vi "uploadSaved.vi"(8 "error in":errorcluster, 11 "Path":path) -> (0 "error out":errorcluster)   [LabVIEW 2024]
uses:
  session.vi
  <vilib>/httpClient/POSTFile.vi
  <vilib>/httpClient/LabVIEWHTTPClient.lvlib
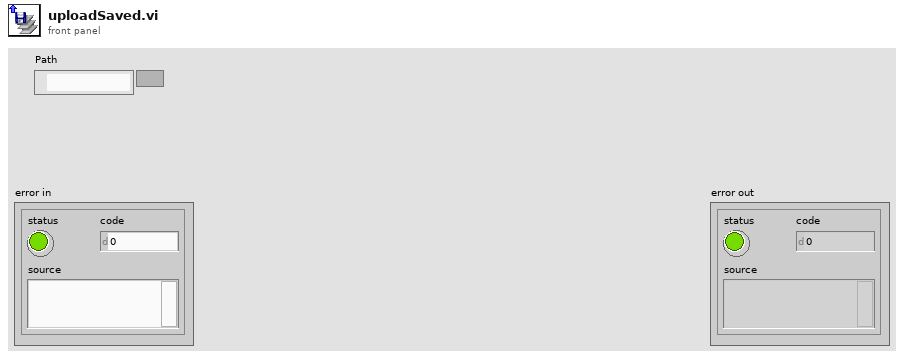
[diagram p1: front panel]
types:
  T1 = typedef "LabVIEWHTTPClient.lvlib/ClientHandle.ctl" = refnum<k1>
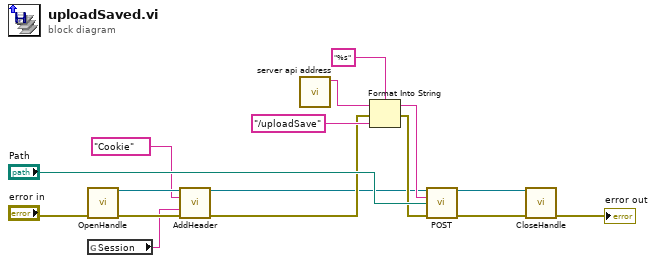
[diagram p0: block diagram]
diagram:
  n1 = call <vilib>:"OpenHandle.vi"("error in (no error)"="error in") -> ("client handle out"=w6:T1, "error out"=w5:errorcluster)  [unwired: 13 in]
  n2 = global read "session.vi" "Session"() -> (w1:string)
  n3 = call <vilib>:"AddHeader.vi"("client handle"=w6, "header"="Cookie", "value"=w1, "error in (no error)"=w5) -> ("client handle out"=w3:T1, "error out"=w4:errorcluster)  [unwired: 10 in]
  n4 = call "server api address.vi"() -> ("Server API URL"=w12:string)  [unwired: 11 in]
  n5 = Format Into String(format string="%s", initial string=w12, error in=w4, "/uploadSave" ("input 1")) -> (resulting string=w14:string, error out=w13:errorcluster)
  n6 = call-poly <vilib>:"POST.vi"("client handle"=w3, "url"=w14, "file"="Path", "error in (no error)"=w13) -> ("client handle out"=w7:T1, "error out"=w8:errorcluster)  [unwired: 8 in, 2 out]
  n7 = call <vilib>:"CloseHandle.vi"("client handle"=w7, "error in (no error)"=w8) -> ("error out"=→"error out":errorcluster)  [unwired: 13 in]
